vi "Loop Status.vi"(8 "error in":errorcluster, 10 "total count":dbl format="%#_6f", 11 "current count":i32) -> (0 "error out":errorcluster, 3 "total count":dbl format="%#_6f")   [LabVIEW 2016]
panel:
  out "Percent Done":dbl(slide) scale=0.0..100.0
  out "current count":i32
  out "Percent Done":dbl
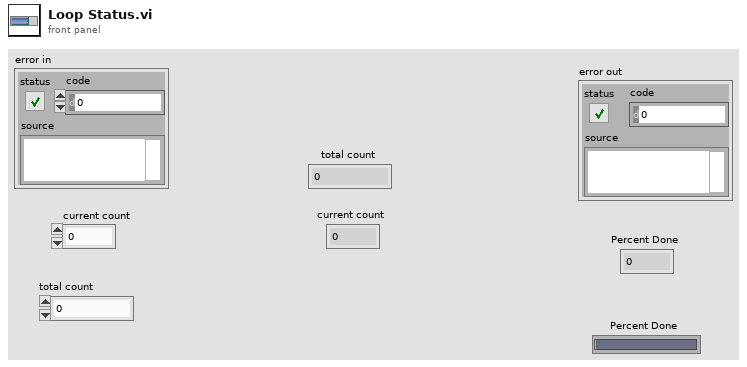
[diagram p1: front panel]
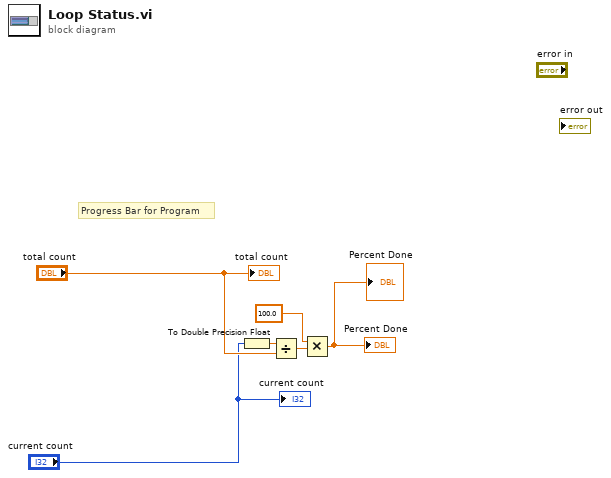
[diagram p0: block diagram]
diagram:
  # "Progress Bar for Program"
  n1 = To Double Precision Float(number="current count") -> (double precision float=w6:dbl)
  n2 = Divide(x=w6, y="total count") -> (x/y=w5:dbl)
  n3 = Multiply(x=100.0, y=w5) -> (x*y=→"Percent Done" →"Percent Done":dbl)
  "total count" <- "total count"
  "current count" <- "current count"
